vi "read_num_elements_from_td.vi"(8 "error in (no error)":errorcluster, 11 "LVData in":refnum<class "LVData.lvclass">) -> (0 "error out":errorcluster, 2 "# elements":u16, 3 "LVData out":refnum<class "LVData.lvclass">)   [LabVIEW 2020, in "lvdata.lvlib" / "LVData.lvclass"]
uses:
  LVData.lvclass
  Bytes/Bytes.lvclass/Bytes.ctl
  2efeb4f9-b79f-4d3e-9f77-c7419c54612c.vi
  2efeb4f9-b79f-4d3e-9f77-c7419c54612c.vi/9518bad7-5904-4cfc-9920-07fa30b29b3b.vi
  Bytes/to_data.vi
  read_type_descriptor.vi
  LVData.lvclass/LVData.ctl
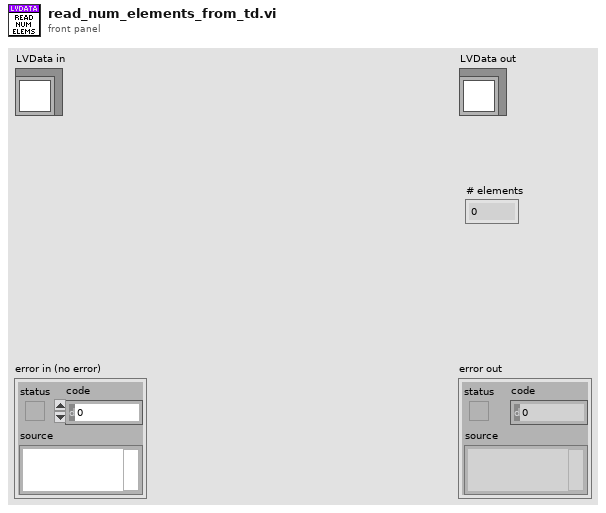
[diagram p1: front panel]
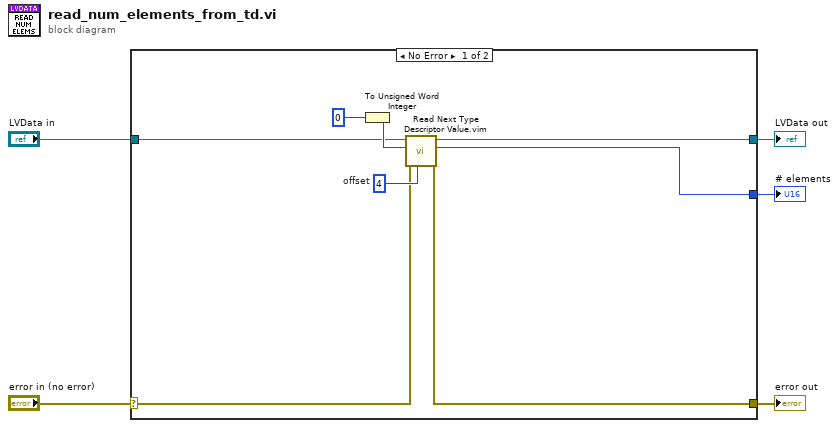
[diagram p0: block diagram]
diagram:
  n1 = case shown="No Error" "error in (no error)" {
    selector: "error in (no error)" -> [w8 w15]
    tunnel: [w7 w15] -> w4
    tunnel: [w10 w14] -> w2
    tunnel: "LVData in" -> [w9 w14]
    tunnel: [w11 _] -> w1
    frame No Error {
      w12 = 4  # offset
      n2 = To Unsigned Word Integer(number=u16 0 ("# elements")) -> (unsigned 16bit integer=w13:u16)
      n3 = call "Read Next Type Descriptor Value.vim"("offset (-1)"=w12, "error in (no error)"=w8, "type"=w13, "LVData in"=w9) -> ("error out"=w7:errorcluster, "value"=w11:u16, "LVData out"=w10:refnum<class "LVData.lvclass">)  [unwired: 5 in]
    }
    frame Error {
    }
  }
  "error out" <- w4
  "LVData out" <- w2
  "# elements" <- w1
